vi "Read_Class_Shielding_Box.vi"(8 "error in (no error)":errorcluster caption="entrée d'erreur (pas d'erreur)", 11 "Class Instrument Multimeter en entrée":refnum<class "Class Instrument Schielding_Box.lvclass">) -> (0 "error out":errorcluster caption="sortie d'erreur", 2 "Class Shielding_ Box":refnum<class "Class Shielding_ Box (Default).lvclass">, 3 "Class Instrument Multimeter en sortie":refnum<class "Class Instrument Schielding_Box.lvclass">)   [LabVIEW 2020, in "Library Instrument & Equipement.lvlib" / "Library Instruments.lvlib" / "Class Instrument Schielding_Box.lvclass"]
uses:
  Class Instrument Schielding_Box.lvclass
  Shielding box/Class Shielding box (Default)/Class Shielding_ Box (Default).lvclass
  Class Instrument Schielding_Box.lvclass/Class Instrument Schielding_Box.ctl
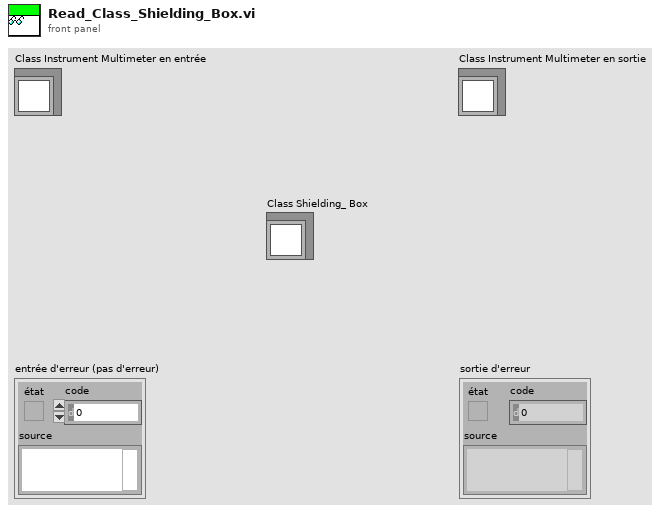
[diagram p1: front panel]
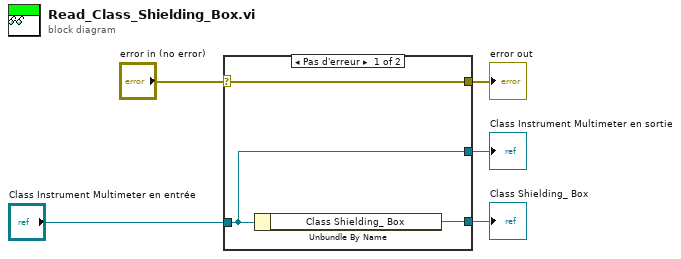
[diagram p0: block diagram]
diagram:
  n1 = case shown="Pas d'erreur" "error in (no error)" {
    selector: "error in (no error)" -> [w8 w9]
    tunnel: [w8 w9] -> w4
    tunnel: [w7 w10] -> w2
    tunnel: "Class Instrument Multimeter en entrée" -> [w7 w10]
    tunnel: [w6 _] -> w1
    frame No Error {
      n2 = Unbundle By Name(w7) -> ("Class Shielding_ Box"=w6:refnum<class "Class Shielding_ Box (Default).lvclass">)
    }
    frame Error {
    }
  }
  "error out" <- w4
  "Class Instrument Multimeter en sortie" <- w2
  "Class Shielding_ Box" <- w1
